vi "UTILITY Aquire Semaphore.vi"(8 "error in (no error)":errorcluster, 10 "Debug":bool, 11 "Refnum in":T1) -> (0 "error out":errorcluster, 3 "Refnum out":T1)   [LabVIEW 2020]
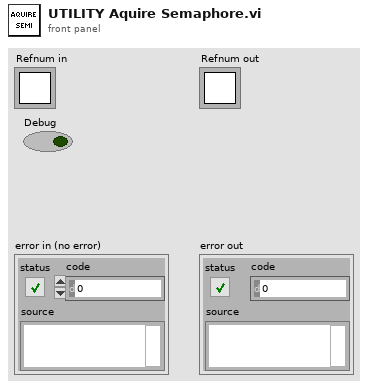
[diagram p1: front panel]
types:
  T1 = typedef "Semaphore RefNum" = refnum<k1>
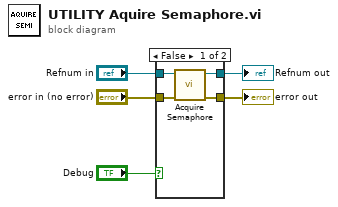
[diagram p0: block diagram]
diagram:
  n1 = case shown="False" "Debug" {
    tunnel: "error in (no error)" -> [w9 w11]
    tunnel: [w8 w11] -> w5
    tunnel: [w7 w10] -> w3
    tunnel: "Refnum in" -> [w6 w10]
    frame False {
      n2 = call <vilib>:"Acquire Semaphore.vi"("error in (no error)"=w9, "semaphore"=w6) -> ("error out"=w8:errorcluster, "semaphore out"=w7:T1)  [unwired: 3 in, 1 out]
    }
    frame True {
    }
  }
  "error out" <- w5
  "Refnum out" <- w3
